vi "Acquisition Message Loop.vi"(8 "error in (no error)":errorcluster, 9 "Data Queue":refnum<queue>, 10 "Data Notifier":refnum<notifier>, 11 "Message Queues":T1) -> (0 "error out":errorcluster)   [LabVIEW 2013, in "Histerese Acquisition.lvlib"]
doc: "Message loop for handling messages pertaining to the acquisition of data from the hardware."
uses:
  Histerese Acquisition.lvlib
  support/Message Queue/All Message Queues.ctl
  support/Message Queue/Message Cluster.ctl
  Hardware Configuration.ctl
  Signal Type.ctl
  Acquisition State.ctl
  support/Message Queue/Enqueue Message (Single).vi
  <vilib>/Utility/error.llb/Error Cluster From Error Code.vi
  <vilib>/ErrorRing/Error Ring.xnode
  support/Message Queue/Histerese Message Queue.lvlib
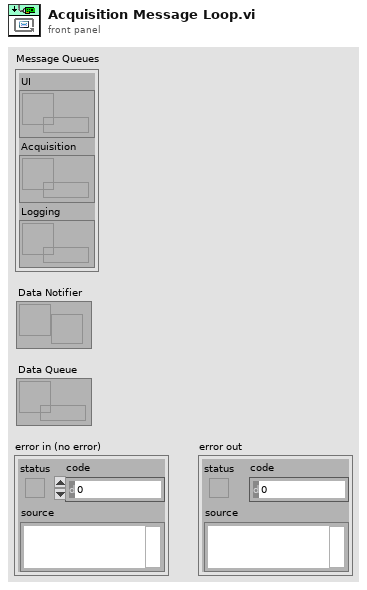
[diagram p1: front panel]
types:
  T1 = typedef "Histerese Message Queue.lvlib/All Message Queues.ctl" = cluster{"UI":refnum<queue>, "Acquisition":refnum<queue>, "Logging":refnum<queue>}
  T2 = typedef "Histerese Acquisition.lvlib/Hardware Configuration.ctl" = cluster{"HW Refnum <Replace Me>":string, "Signal Type <Replace Me>":T3}
  T3 = typedef "Histerese Acquisition.lvlib/Signal Type.ctl" = enum16{"Sine Wave", "Square with Noise"}
  T4 = typedef "Histerese Acquisition.lvlib/Acquisition State.ctl" = enum16{"Idle", "Acquiring"}
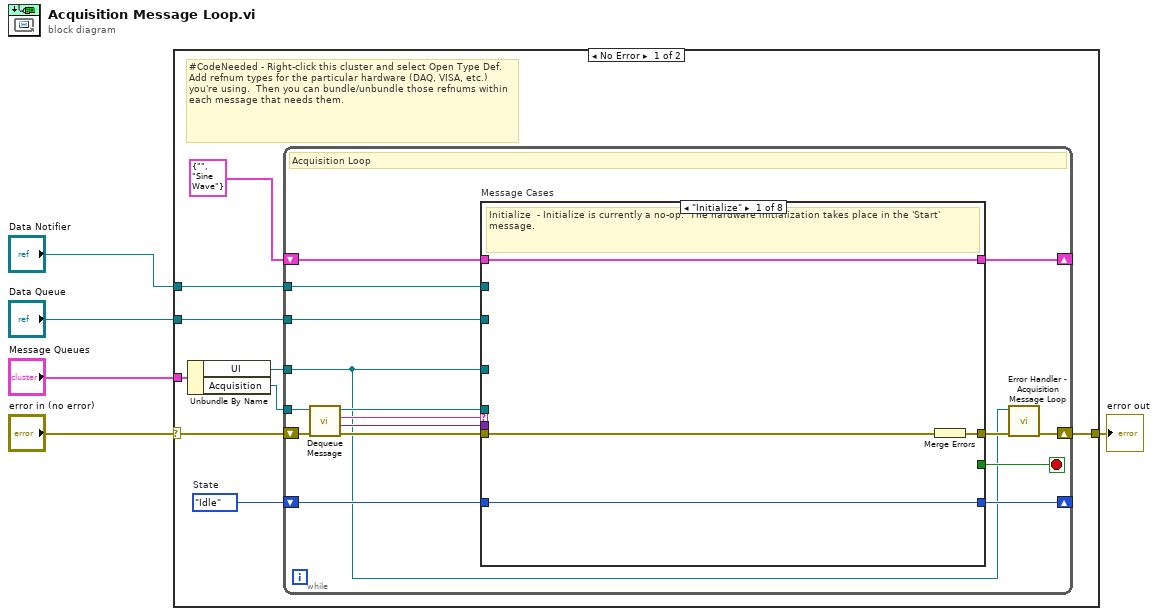
[diagram p0: block diagram]
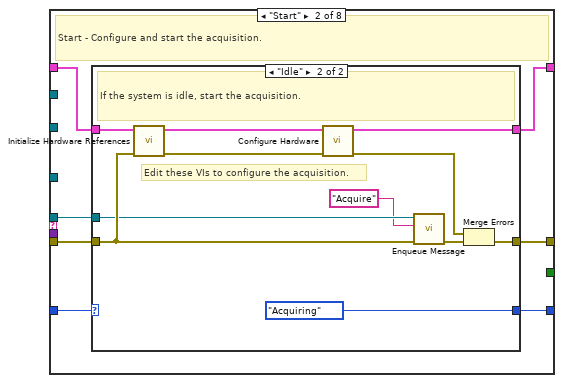
[diagram p2: hidden frame]
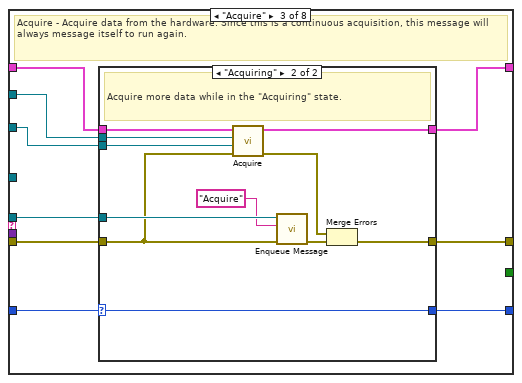
[diagram p4: hidden frame]
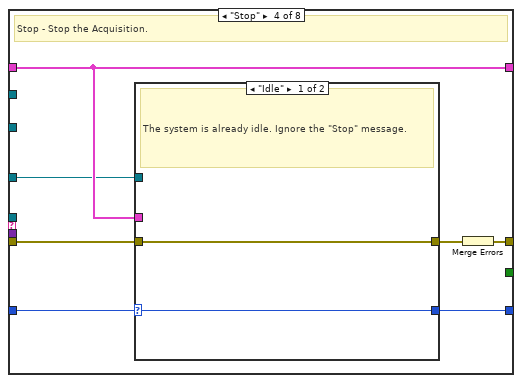
[diagram p6: hidden frame]
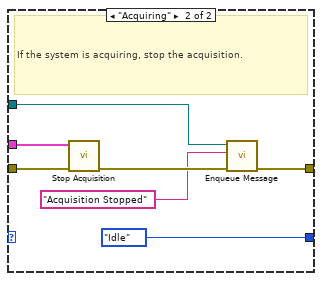
[diagram p7: hidden frame]
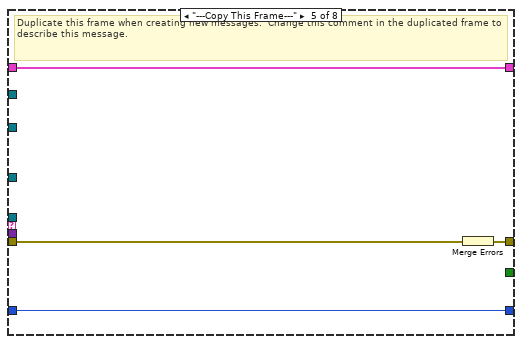
[diagram p8: hidden frame]
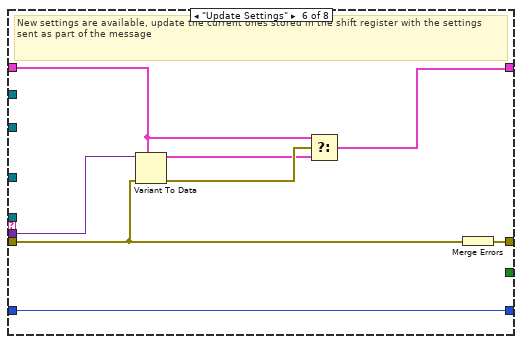
[diagram p9: hidden frame]
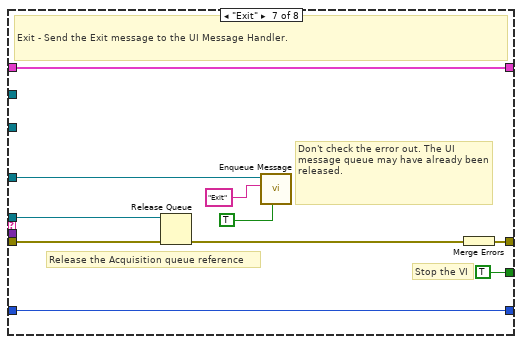
[diagram p10: hidden frame]
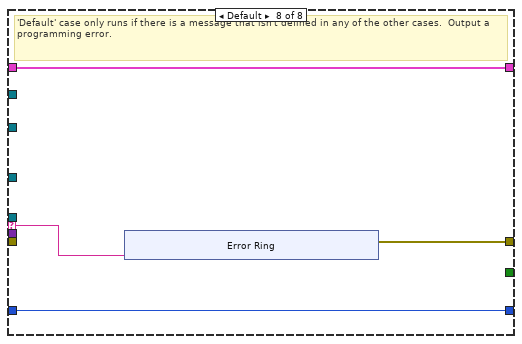
[diagram p11: hidden frame]
diagram:
  n1 = case shown="No Error" "error in (no error)" {
    selector: "error in (no error)" -> [w10 w128]
    tunnel: "Message Queues" -> [w14 _]
    tunnel: [w12 w128] -> w4
    tunnel: "Data Notifier" -> [w8 _]
    tunnel: "Data Queue" -> [w7 _]
    frame No Error {
      w6 = Acquisition_State."Idle"  # State
      # "#CodeNeeded - Right-click this cluster and select Open Type Def.  Add refnum types for the particular hardware (DAQ, VISA, etc.) you're using.  Then you can bundle/unbundle those refnums within each message that needs them."
      n2 = Unbundle By Name(w14) -> ("UI"=w9:refnum<queue>, "Acquisition"=w13:refnum<queue>)
      n3 = while {
        tunnel: w13 -> [w23]
        shift-right: [w29] -> _
        shift-left: T2 {"HW Refnum <Replace Me>"="", "Signal Type <Replace Me>"=enum."Sine Wave"} ("Data Cluster") -> [w30]
        shift-right: [w18] -> w12
        shift-left: w10 -> [w27]
        tunnel: w9 -> [w15]
        tunnel: w8 -> [w22]
        tunnel: w7 -> [w21]
        shift-right: [w19] -> _
        shift-left: w6 -> [w20]
        stop <- w28 stop-if-true
        # "Acquisition Loop"
        n4 = call "Dequeue Message.vi"("error in (no error)"=w27, "Message Queue"=w23) -> ("error out"=w26:errorcluster, "Message Data"=w24:variant, "Message"=w25:string, "dup Message Queue"=w16:refnum<queue>)  [unwired: 6 in]
        n5 = case "Message Cases" shown="\"Initialize\"" w25 {
          selector: w25 -> [_ _ _ _ _ _ _ w117]
          tunnel: w16 -> [_ w38 w63 _ _ _ w108 _]
          tunnel: w26 -> [w33 w39 w62 w84 w98 w100 w112 _]
          tunnel: [w34 w41 w64 w85 w96 w106 w115 w118] -> w17
          tunnel: w30 -> [w32 w40 w60 w82 w97 w102 w114 w120]
          tunnel: [w32 w37 w61 w82 w97 w101 w114 w120] -> w29
          tunnel: [_ _ _ _ _ _ TRUE _] -> w28
          tunnel: w24 -> [_ _ _ _ _ w105 _ _]
          tunnel: w15 -> [_ _ _ w79 _ _ w113 _]
          tunnel: w22 -> [_ _ w59 _ _ _ _ _]
          tunnel: w21 -> [_ _ w58 _ _ _ _ _]
          tunnel: w20 -> [w31 w35 w56 w81 w95 w99 w107 w119]
          tunnel: [w31 w36 w57 w80 w95 w99 w107 w119] -> w19
          frame "Initialize" {
            # "Initialize  - Initialize is currently a no-op.  The hardware initialization takes place in the 'Start' message."
            n6 = Merge Errors(w33) -> (w34:errorcluster)
          }
          frame "Start" {
            # "Start - Configure and start the acquisition."
            n7 = case shown="\"Idle\"" w35 {
              selector: w35 -> [w42 _]
              tunnel: [w43 w55] -> w41
              tunnel: w40 -> [w44 w54]
              tunnel: w39 -> [w43 w53]
              tunnel: w38 -> [_ w51]
              tunnel: [w44 w47] -> w37
              tunnel: [w42 Acquisition_State."Acquiring" ("Acquisition State")] -> w36
              frame "Acquiring" {
                # "The system is already acquiring. Ignore the \"Start\" message."
              }
              frame "Idle" {
                # "Edit these VIs to configure the acquisition."
                # "If the system is idle, start the acquisition."
                n8 = call "Initialize Hardware References.vi"("error in (no error)"=w53, "Hardware Resources in"=w54) -> ("error out"=w50:errorcluster, "Hardware Resources out"=w48:T2)  [unwired: 8 in]
                n9 = call "Configure Hardware.vi"("error in (no error)"=w50, "Hardware Resources in"=w48) -> ("error out"=w49:errorcluster, "Hardware Resources out"=w47:T2)  [unwired: 8 in]
                n10 = call-poly "Enqueue Message.vi"("error in (no error)"=w53, "Message"="Acquire", "Message Queue"=w51) -> ("error out"=w52:errorcluster)  [unwired: 7 in, 1 out]
                n11 = Merge Errors(w49, w52) -> (w55:errorcluster)
              }
            }
          }
          frame "Acquire" {
            # "Acquire - Acquire data from the hardware. Since this is a continuous acquisition, this message will always message itself to run again."
            n12 = case shown="\"Acquiring\"" w56 {
              selector: w56 -> [w65 w69]
              tunnel: [w66 w78] -> w64
              tunnel: w63 -> [_ w76]
              tunnel: w62 -> [w66 w68]
              tunnel: [w67 w74] -> w61
              tunnel: w60 -> [w67 w73]
              tunnel: w59 -> [_ w71]
              tunnel: w58 -> [_ w70]
              tunnel: [w65 w69] -> w57
              frame "Idle" {
                # "Ignore \"Acquire\" messages when the acquisition is idle."
              }
              frame "Acquiring" {
                # "Acquire more data while in the \"Acquiring\" state."
                n13 = call "Acquire.vi"("error in (no error)"=w68, "Data Queue"=w70, "Data Notifier"=w71, "Hardware Resources in"=w73) -> ("error out"=w75:errorcluster, "Hardware Resources out"=w74:T2)  [unwired: 6 in]
                n14 = call-poly "Enqueue Message.vi"("error in (no error)"=w68, "Message"="Acquire", "Message Queue"=w76) -> ("error out"=w77:errorcluster)  [unwired: 7 in, 1 out]
                n15 = Merge Errors(w75, w77) -> (w78:errorcluster)
              }
            }
          }
          frame "Stop" {
            # "Stop - Stop the Acquisition."
            n16 = case shown="\"Idle\"" w81 {
              selector: w81 -> [w86 _]
              tunnel: w84 -> [w87 w94]
              tunnel: [w87 w90] -> w83
              tunnel: w82 -> [_ w92]
              tunnel: [w86 Acquisition_State."Idle" ("State")] -> w80
              tunnel: w79 -> [_ w89]
              frame "Idle" {
                # "The system is already idle. Ignore the \"Stop\" message."
              }
              frame "Acquiring" {
                # "If the system is acquiring, stop the acquisition."
                n17 = call "Stop Acquisition.vi"("error in (no error)"=w94, "Hardware Resources in"=w92) -> ("error out"=w93:errorcluster)  [unwired: 9 in]
                n18 = call-poly "Enqueue Message.vi"("error in (no error)"=w93, "Message"="Acquisition Stopped", "Message Queue"=w89) -> ("error out"=w90:errorcluster)  [unwired: 7 in, 1 out]
              }
            }
            n19 = Merge Errors(w83) -> (w85:errorcluster)
          }
          frame "---Copy This Frame---" {
            # "Duplicate this frame when creating new messages.  Change this comment in the duplicated frame to describe this message."
            n20 = Merge Errors(w98) -> (w96:errorcluster)
          }
          frame "Update Settings" {
            # "New settings are available, update the current ones stored in the shift register with the settings sent as part of the message"
            n21 = Variant To Data(error in=w100, type=w102, Variant=w105) -> (data=w103:T2, error out=w104:errorcluster)
            n22 = Select(t=w102, s=w104, f=w103) -> (s? t:f=w101:T2)
            n23 = Merge Errors(w100) -> (w106:errorcluster)
          }
          frame "Exit" {
            # "Don't check the error out. The UI message queue may have already been released."
            # "Release the Acquisition queue reference"
            # "Stop the VI"
            # "Exit - Send the Exit message to the UI Message Handler."
            n24 = Release Queue(queue=w108, error in (no error)=w112) -> (error out=w109:errorcluster)  [unwired: 1 in, 2 out]
            n25 = call-poly "Enqueue Message.vi"("Priority Message? (F)"=TRUE, "Message"="Exit", "Message Queue"=w113) -> ()  [unwired: 7 in, 2 out]
            n26 = Merge Errors(w109) -> (w115:errorcluster)
          }
          frame Default {
            # "'Default' case only runs if there is a message that isn't defined in any of the other cases.  Output a programming error."
            n27 = xnode "Error Ring"("parameter 0"=w117) -> ("error out"=w118:errorcluster)
          }
        }
        n28 = call "Error Handler - Acquisition Message Loop.vi"("error in (no error)"=w17, "Message Queue"=w15) -> ("dup error in"=w18:errorcluster)  [unwired: 8 in, 1 out]
      }
    }
    frame Error {
    }
  }
  "error out" <- w4
